vi "Random_Pts.vi"(1 "Num of Points":i32, 2 "z bound":dbl, 3 "y bound":dbl, 4 "x bound":dbl) -> (0 "appended array":dbl[][](array[numeric]))   [LabVIEW 2019]
uses:
  <vilib>/numeric/Random Number (Range) DBL.vi
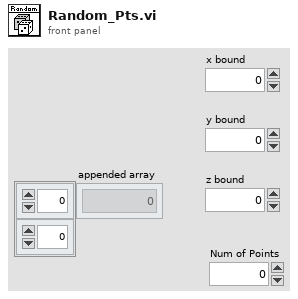
[diagram p1: front panel]
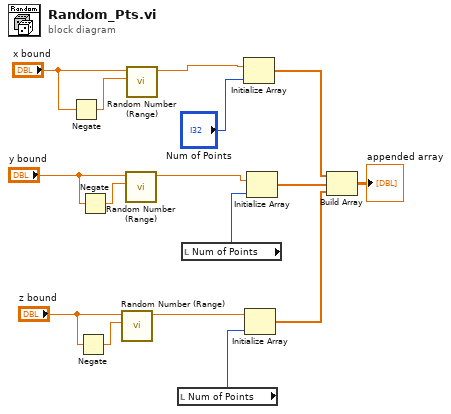
[diagram p0: block diagram]
diagram:
  n1 = Negate(x="x bound") -> (-x=w15:dbl)
  n2 = Negate(x="z bound") -> (-x=w12:dbl)
  n3 = Negate(x="y bound") -> (-x=w14:dbl)
  n4 = call-poly <vilib>:"Random Number (Range).vi"("lower bound (0)"=w12, "upper bound (100)"="z bound") -> ("number"=w8:dbl)  [unwired: 9 in]
  n5 = call-poly <vilib>:"Random Number (Range).vi"("lower bound (0)"=w14, "upper bound (100)"="y bound") -> ("number"=w9:dbl)  [unwired: 9 in]
  n6 = call-poly <vilib>:"Random Number (Range).vi"("lower bound (0)"=w15, "upper bound (100)"="x bound") -> ("number"=w10:dbl)  [unwired: 9 in]
  n7 = local read "Num of Points"() -> (w2:i32)
  n8 = local read "Num of Points"() -> (w3:i32)
  n9 = Initialize Array(w10, "Num of Points") -> (w7:dbl[])
  n10 = Initialize Array(w8, w2) -> (w5:dbl[])
  n11 = Initialize Array(w9, w3) -> (w6:dbl[])
  n12 = Build Array(w7, w6, w5) -> (→"appended array":dbl[][])
